vi "KE622x -- 2182 -A A Read-Out Loop.vi"(0 "622x Resource In":refnum<visa-resource-name>, 1 "Check For SCPI Errors? (T)":bool=TRUE, 7 "Time of one measurement":dbl=1000.0 min=0.0, 11 "error in (no error)":errorcluster) -> (4 "622x Resource Out (dupl)":refnum<visa-resource-name>, 8 "2182-A Reponse String":string, 15 "error out":errorcluster)   [LabVIEW 2013, in "Keithly user program.lvlib"]
doc: "Return measured value from instrument KE2182-A."
uses:
  Keithly user program.lvlib
panel:
  in  "y":bool
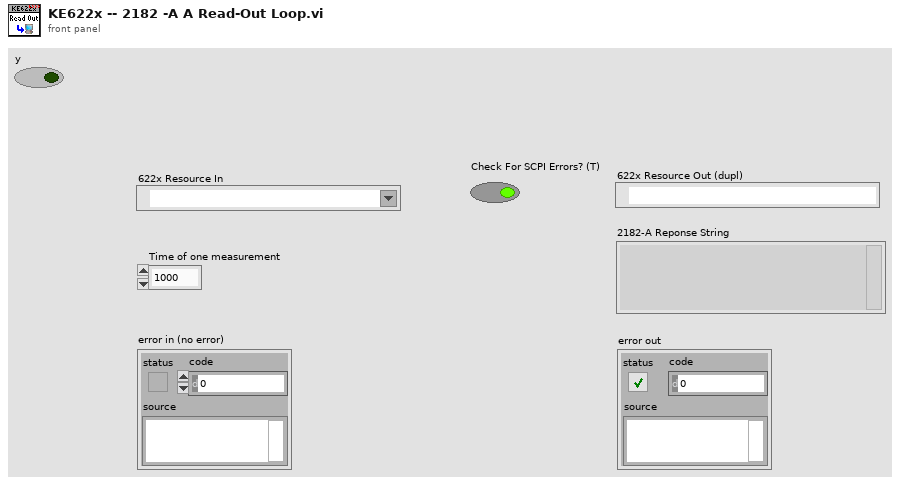
[diagram p1: front panel]
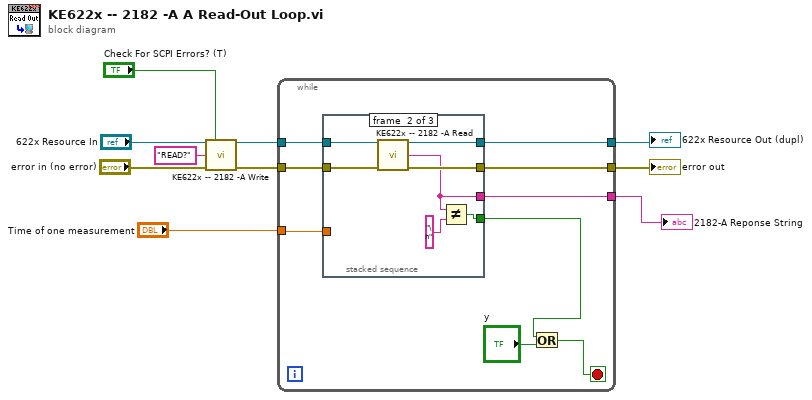
[diagram p0: block diagram]
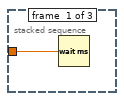
[diagram p2: hidden frame]
diagram:
  n1 = call "KE622x -- 2182 -A Write.vi"("Resource In"="622x Resource In", "Check For SCPI Errors? (T)"="Check For SCPI Errors? (T)", "2182-A Write String"="READ?", "error in (no error)"="error in (no error)") -> ("Resource Out (dupl)"=w6:refnum<visa-resource-name>, "error out"=w5:errorcluster)  [unwired: 10 in]
  n2 = while {
    tunnel: w6 -> [w19]
    tunnel: w5 -> [w18]
    tunnel: "Time of one measurement" -> [w17]
    tunnel: [w16] -> w2
    tunnel: [w15] -> w1
    tunnel: [w11] -> w4
    stop <- w14 stop-if-true
    n3 = stacked-sequence {
      tunnel: w19 -> [_ w27 _]
      tunnel: w18 -> [_ w26 _]
      tunnel: w17 -> [w20 _ _]
      tunnel: [_ w25 _] -> w16
      tunnel: [_ w24 _] -> w15
      tunnel: [_ w22 _] -> w12
      tunnel: [_ w21 _] -> w11
      frame #0 {
        n4 = Wait (ms)(milliseconds to wait=w20) -> ()  [unwired: 1 out]
      }
      frame #1 {
        n5 = call "KE622x -- 2182 -A Read.vi"("622x Resource In"=w27, "error in (no error)"=w26) -> ("622x Resource Out (dupl)"=w25:refnum<visa-resource-name>, "2182-A Reponse String"=w21:string, "error out"=w24:errorcluster)  [unwired: 11 in]
        n6 = Not Equal?(x=w21, y="\n") -> (x != y?=w22:bool)
      }
      frame #2 {
      }
    }
    n7 = Or(x=w12, y="y") -> (x .or. y?=w14:bool)
  }
  "622x Resource Out (dupl)" <- w2
  "error out" <- w1
  "2182-A Reponse String" <- w4
